vi "New.vi"(7 "Endianess":T1, 8 "error in (no error)":errorcluster, 9 "Buffer Size (#timestamps)":i32, 10 "Size(s)":i32[](array[numeric]), 11 "Data Type":T2) -> (0 "error out":errorcluster, 3 "Ring Buffer":T3)   [LabVIEW 2021, in "Ring Buffer Strict Accessor.lvlib"]
uses:
  Ring Buffer Strict Accessor.lvlib
  SubVIs/RingBufferHandle.ctl
  <userlib>/bjustice/Ring Buffer for Time Series Data/SubVIs/DVR data.ctl
  SubVIs/DataType.ctl
  SubVIs/Endianess.ctl
  <vilib>/Utility/error.llb/whitespace.ctl
  <vilib>/Utility/error.llb/Error Cluster From Error Code.vi
  <vilib>/ErrorRing/Error Ring.xnode
  <userlib>/bjustice/Ring Buffer for Time Series Data/Ring Buffer Time Series Data.lvlib
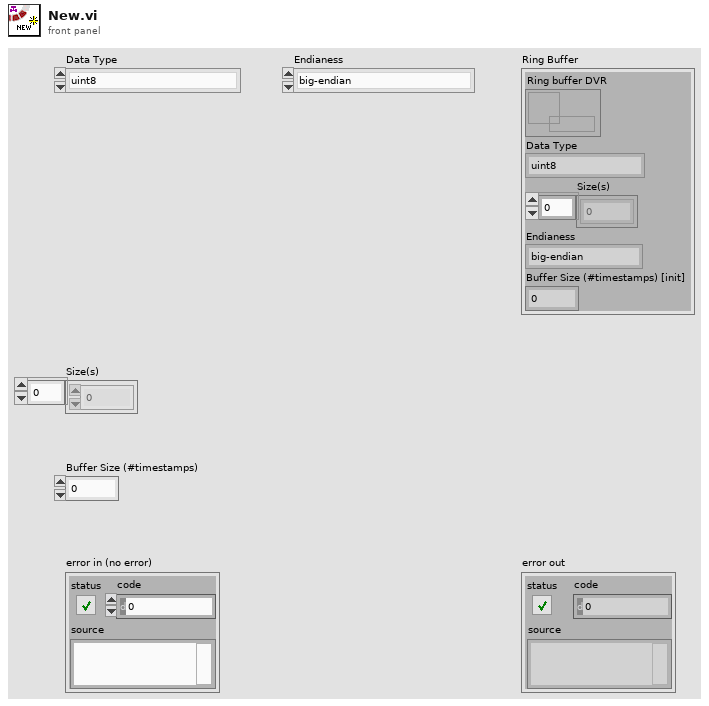
[diagram p1: front panel]
types:
  T1 = typedef "Ring Buffer Strict Accessor.lvlib/Endianess.ctl" = enum16{"big-endian", "little-endian"}
  T2 = typedef "Ring Buffer Strict Accessor.lvlib/DataType.ctl" = enum16{"uint8", "uint16", "uint32", "uint64", "int8", "int16", "int32", "int64", "float", "double", "extended"}
  T3 = typedef "Ring Buffer Strict Accessor.lvlib/RingBufferHandle.ctl" = cluster{"Ring buffer DVR":refnum<data-value>, "Data Type":T2, "Size(s)":i32[], "Endianess":T1, "Buffer Size (#timestamps) [init]":i32}
  T4 = typedef "whitespace.ctl" = u16
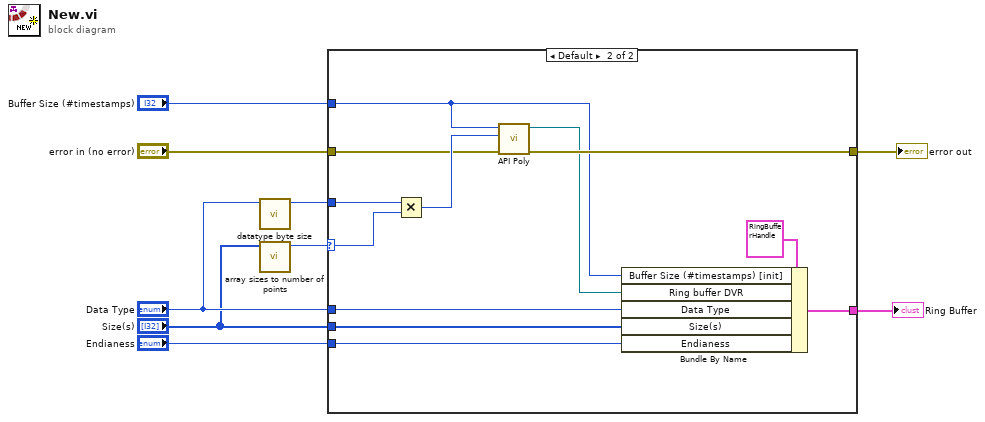
[diagram p0: block diagram]
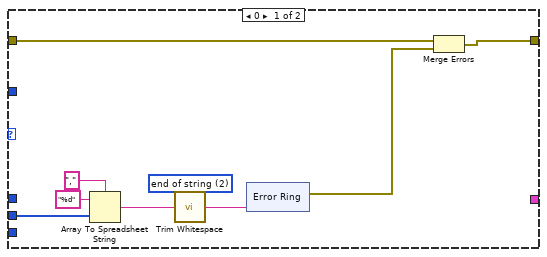
[diagram p2: hidden frame]
diagram:
  n1 = call "datatype byte size.vi"("Data Type"="Data Type") -> ("#bytes per scalar value"=w3:i32)  [unwired: 10 in]
  n2 = call "array sizes to number of points.vi"("Size(s)"="Size(s)") -> ("#scalar values"=w1:i32)  [unwired: 10 in]
  n3 = case shown="Default" w1 {
    selector: w1 -> [_ w28]
    tunnel: [_ w36] -> w9
    tunnel: "Endianess" -> [_ w35]
    tunnel: "Buffer Size (#timestamps)" -> [_ w27]
    tunnel: "error in (no error)" -> [w12 w33]
    tunnel: [w10 w32] -> w5
    tunnel: "Data Type" -> [_ w31]
    tunnel: w3 -> [_ w30]
    tunnel: "Size(s)" -> [w14 w29]
    frame 0 {
      w15 = T4 2 items=["both", "start of string", "end of string"] ("location (both)")
      n4 = Array To Spreadsheet String(delimiter (Tab)=",", array=w14, 3:"%d" ("format string")) -> (spreadsheet string=w16:string)
      n5 = call <vilib>:"Trim Whitespace.vi"("string"=w16, "location (both)"=w15) -> ("trimmed string"=w13:string)
      n6 = xnode "Error Ring"("parameter 0"=w13) -> ("error out"=w11:errorcluster)
      n7 = Merge Errors(w12, w11) -> (w10:errorcluster)
    }
    frame Default {
      n8 = Multiply(x=w30, y=w28) -> (x*y=w34:i32)
      n9 = call-poly <userlib>:"API Poly.vi"("error in (no error)"=w33, "#bytes per timestamp"=w34, "Buffer Size (#timestamps)"=w27) -> ("error out"=w32:errorcluster, "Ring buffer DVR"=w26:refnum<data-value>)  [unwired: 7 in]
      n10 = Bundle By Name(cluster=T3 {"Ring buffer DVR"=refnum, "Data Type"=enum."uint8", "Size(s)"=[], "Endianess"=enum."big-endian", "Buffer Size (#timestamps) [init]"=0} ("value (Add)"), "Buffer Size (#timestamps) [init]"=w27, "Ring buffer DVR"=w26, "Data Type"=w31, "Size(s)"=w29, "Endianess"=w35) -> (w36:T3)
    }
  }
  "Ring Buffer" <- w9
  "error out" <- w5
